vi "register_swabian_events.vi"(8 "error in (no error)":errorcluster) -> (0 "error out":errorcluster, 2 "events":T2, 3 "references":T1)   [LabVIEW 2018]
uses:
  swabian_events_tdef.ctl
  update_chart_tdef.ctl
  channel_data_tdef.ctl
  swabian_event_refs.ctl
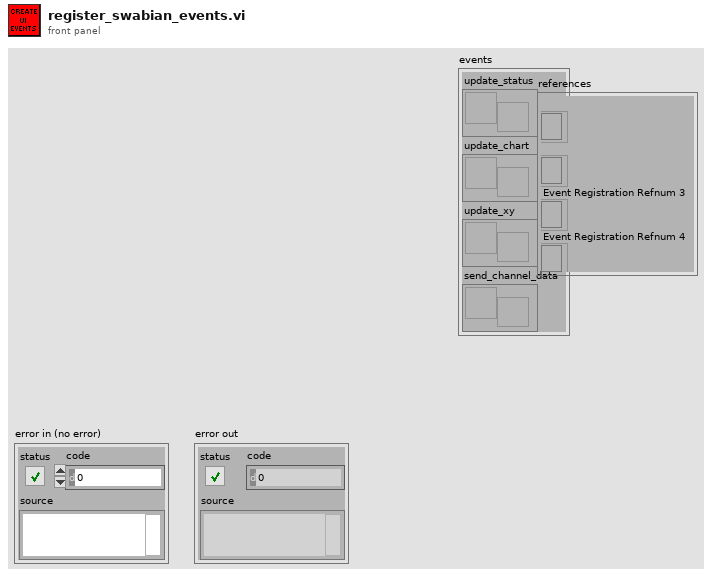
[diagram p1: front panel]
types:
  T1 = typedef "swabian_event_refs.ctl" = cluster{"event registration refnum":refnum<event-registration>, "Event Registration Refnum 2":refnum<event-registration>, "Event Registration Refnum 3":refnum<event-registration>, "Event Registration Refnum 4":refnum<event-registration>}
  T2 = typedef "swabian_events_tdef.ctl" = cluster{"update_status":refnum<user-event>, "update_chart":refnum<user-event>, "update_xy":refnum<user-event>, "send_channel_data":refnum<user-event>}
  T3 = typedef "channel_data_tdef.ctl" = cluster{"data":cluster{dbl[], dbl[]}, "channel":u8}
  T4 = typedef "update_chart_tdef.ctl" = cluster{"ch0":dbl, "ch1":dbl, "ch2":dbl, "ch3":dbl, "ch4":dbl, "ch5":dbl, "ch6":dbl, "ch7":dbl}
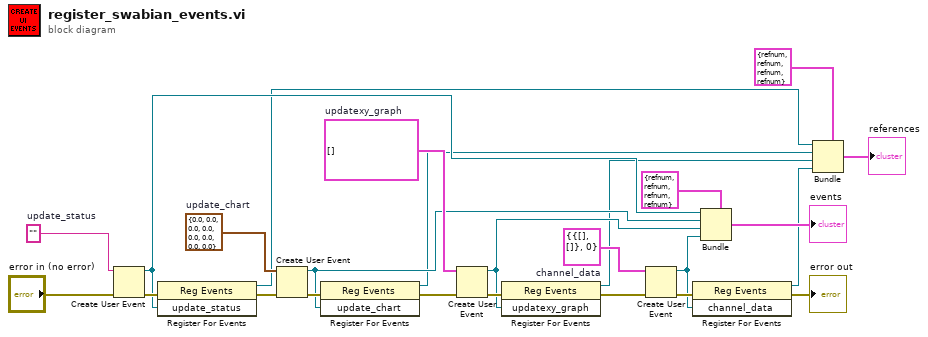
[diagram p0: block diagram]
diagram:
  w13 = T3 {"data"={[], []}, "channel"=0}  # channel_data
  w14 = cluster{dbl[], dbl[]}[] []  # updatexy_graph
  w22 = T4 {"ch0"=0.0, "ch1"=0.0, "ch2"=0.0, "ch3"=0.0, "ch4"=0.0, "ch5"=0.0, "ch6"=0.0, "ch7"=0.0}  # update_chart
  w25 = ""  # update_status
  n1 = Create User Event(user event datatype=w25, error in="error in (no error)") -> (user event=w9:refnum<user-event>, error out=w23:errorcluster)
  n2 = register-events(error in=w23, w9) -> (reference out=w4:refnum<event-registration>, error out=w5:errorcluster)  [unwired: 1 in]
  n3 = Create User Event(user event datatype=w22, error in=w5) -> (user event=w8:refnum<user-event>, error out=w19:errorcluster)
  n4 = register-events(error in=w19, w8) -> (reference out=w3:refnum<event-registration>, error out=w16:errorcluster)  [unwired: 1 in]
  n5 = Create User Event(user event datatype=w14, error in=w16) -> (user event=w7:refnum<user-event>, error out=w15:errorcluster)
  n6 = register-events(error in=w15, w7) -> (reference out=w2:refnum<event-registration>, error out=w12:errorcluster)  [unwired: 1 in]
  n7 = Create User Event(user event datatype=w13, error in=w12) -> (user event=w6:refnum<user-event>, error out=w11:errorcluster)
  n8 = register-events(error in=w11, w6) -> (reference out=w1:refnum<event-registration>, error out=→"error out":errorcluster)  [unwired: 1 in]
  n9 = Bundle(cluster=T2 {"update_status"=refnum, "update_chart"=refnum, "update_xy"=refnum, "send_channel_data"=refnum} ("output cluster"), "update_status"=w9, "update_chart"=w8, "update_xy"=w7, "send_channel_data"=w6) -> (→"events":T2)
  n10 = Bundle(cluster=T1 {"event registration refnum"=refnum, "Event Registration Refnum 2"=refnum, "Event Registration Refnum 3"=refnum, "Event Registration Refnum 4"=refnum} ("output cluster"), "event registration refnum"=w4, "Event Registration Refnum 2"=w3, "Event Registration Refnum 3"=w2, "Event Registration Refnum 4"=w1) -> (→"references":T1)
